vi "SetData.vi"(7 "LabVIEW Web Service Request":refnum<class "Web Request.lvclass">) -> ()   [LabVIEW 2014]
uses:
  <vilib>/wsapi/Web Request.lvclass
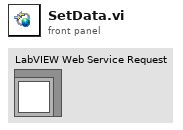
[diagram p1: front panel]
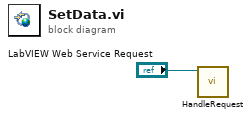
[diagram p0: block diagram]
diagram:
  n1 = call "HandleRequest.vi"("Web Request in"="LabVIEW Web Service Request") -> ()  [unwired: 9 in, 2 out]
